vi "Get_Mean_A+P.vi"(5 "Wait [s]":dbl, 6 "Frequency [Hz]":dbl, 7 "error in (no error)":errorcluster) -> (0 "Mean Amplitude":dbl, 1 "Error Amplitude":dbl, 2 "Mean Phase Shift":dbl, 3 "error out":errorcluster, 4 "Error Phase Shift":dbl)   [LabVIEW 2010]
uses:
  <vilib>/Analysis/NI_AALBase.lvlib
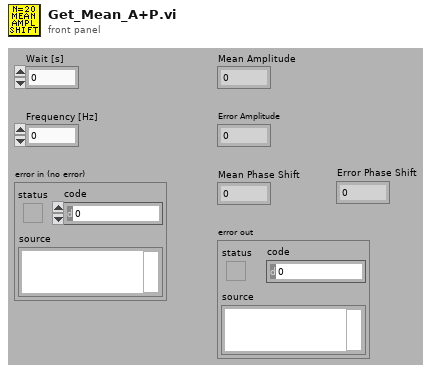
[diagram p1: front panel]
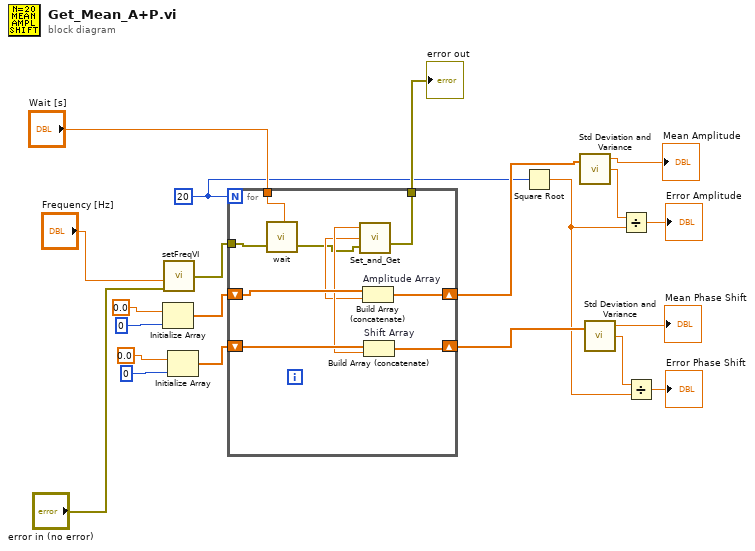
[diagram p0: block diagram]
diagram:
  w10 = 20
  n1 = Initialize Array(0.0, 0) -> (w6:dbl[])
  n2 = call "setFreqVI.vi"("error in"="error in (no error)", "Frequenz in Hz"="Frequency [Hz]") -> ("error out"=w8:errorcluster)  [unwired: 2 in]
  n3 = Initialize Array(0.0, 0) -> (w1:dbl[])
  n4 = for {
    N: w10 -> [_]
    tunnel: w8 -> [w22]
    shift-right: [w28] -> w13
    shift-left: w1 -> [w29]
    shift-right: [w31] -> w20
    shift-left: w6 -> [w30]
    tunnel: [w25] -> w11
    tunnel: "Wait [s]" -> [w23]
    n5 = call "wait.vi"("error in"=w22, "Wartezeit in Sek"=w23) -> ("error out"=w24:errorcluster)  [unwired: 1 in]
    n6 = call "Set_and_Get.vi"("error in (no error)"=w24) -> ("error out"=w25:errorcluster, "Amplitude"=w26:dbl, "Phase Shift"=w27:dbl)  [unwired: 1 in]
    n7 = Build Array (concatenate) "Amplitude Array"(w30, w26) -> (w31:dbl[])
    n8 = Build Array (concatenate) "Shift Array"(w29, w27) -> (w28:dbl[])
  }
  "error out" <- w11
  n9 = Square Root(x=w10) -> (sqrt(x)=w12:dbl)
  n10 = call <vilib>:"Std Deviation and Variance.vi"("X"=w20) -> ("mean"=→"Mean Amplitude":dbl, "standard deviation"=w17:dbl)  [unwired: 1 in, 1 out]
  n11 = call <vilib>:"Std Deviation and Variance.vi"("X"=w13) -> ("mean"=→"Mean Phase Shift":dbl, "standard deviation"=w16:dbl)  [unwired: 1 in, 1 out]
  n12 = Divide(x=w17, y=w12) -> (x/y=→"Error Amplitude":dbl)
  n13 = Divide(x=w16, y=w12) -> (x/y=→"Error Phase Shift":dbl)
